vi "GC Vacuum - Step 8.vi"(7 "Step":i32, 8 "error in":errorcluster, 9 "Test Results In":T8, 10 "Gas":T1, 11 "GC Configuration":T2) -> (0 "error out":errorcluster, 1 "Test Results Out":T8, 2 "Gas Out":T1 caption="Gas", 3 "GC Configuration Out":T2)   [LabVIEW 2015]
uses:
  Controls/Test Information.ctl
  Controls/Vacuum Test.ctl
  Controls/Test Timing.ctl
  Controls/Vaccum Thresholds.ctl
  Controls/Helium Test.ctl
  Controls/Helium Thresholds.ctl
  CAN Communication/Gas/Typedefs/Session Handle.ctl
  CAN Communication/Gas/Gas.lvclass
  Controls/Test Results.ctl
  Controls/Step Result.ctl
  CAN Communication/Gas/Typedefs/Valves.ctl
  SubVIs/Timing/Timing.lvlib
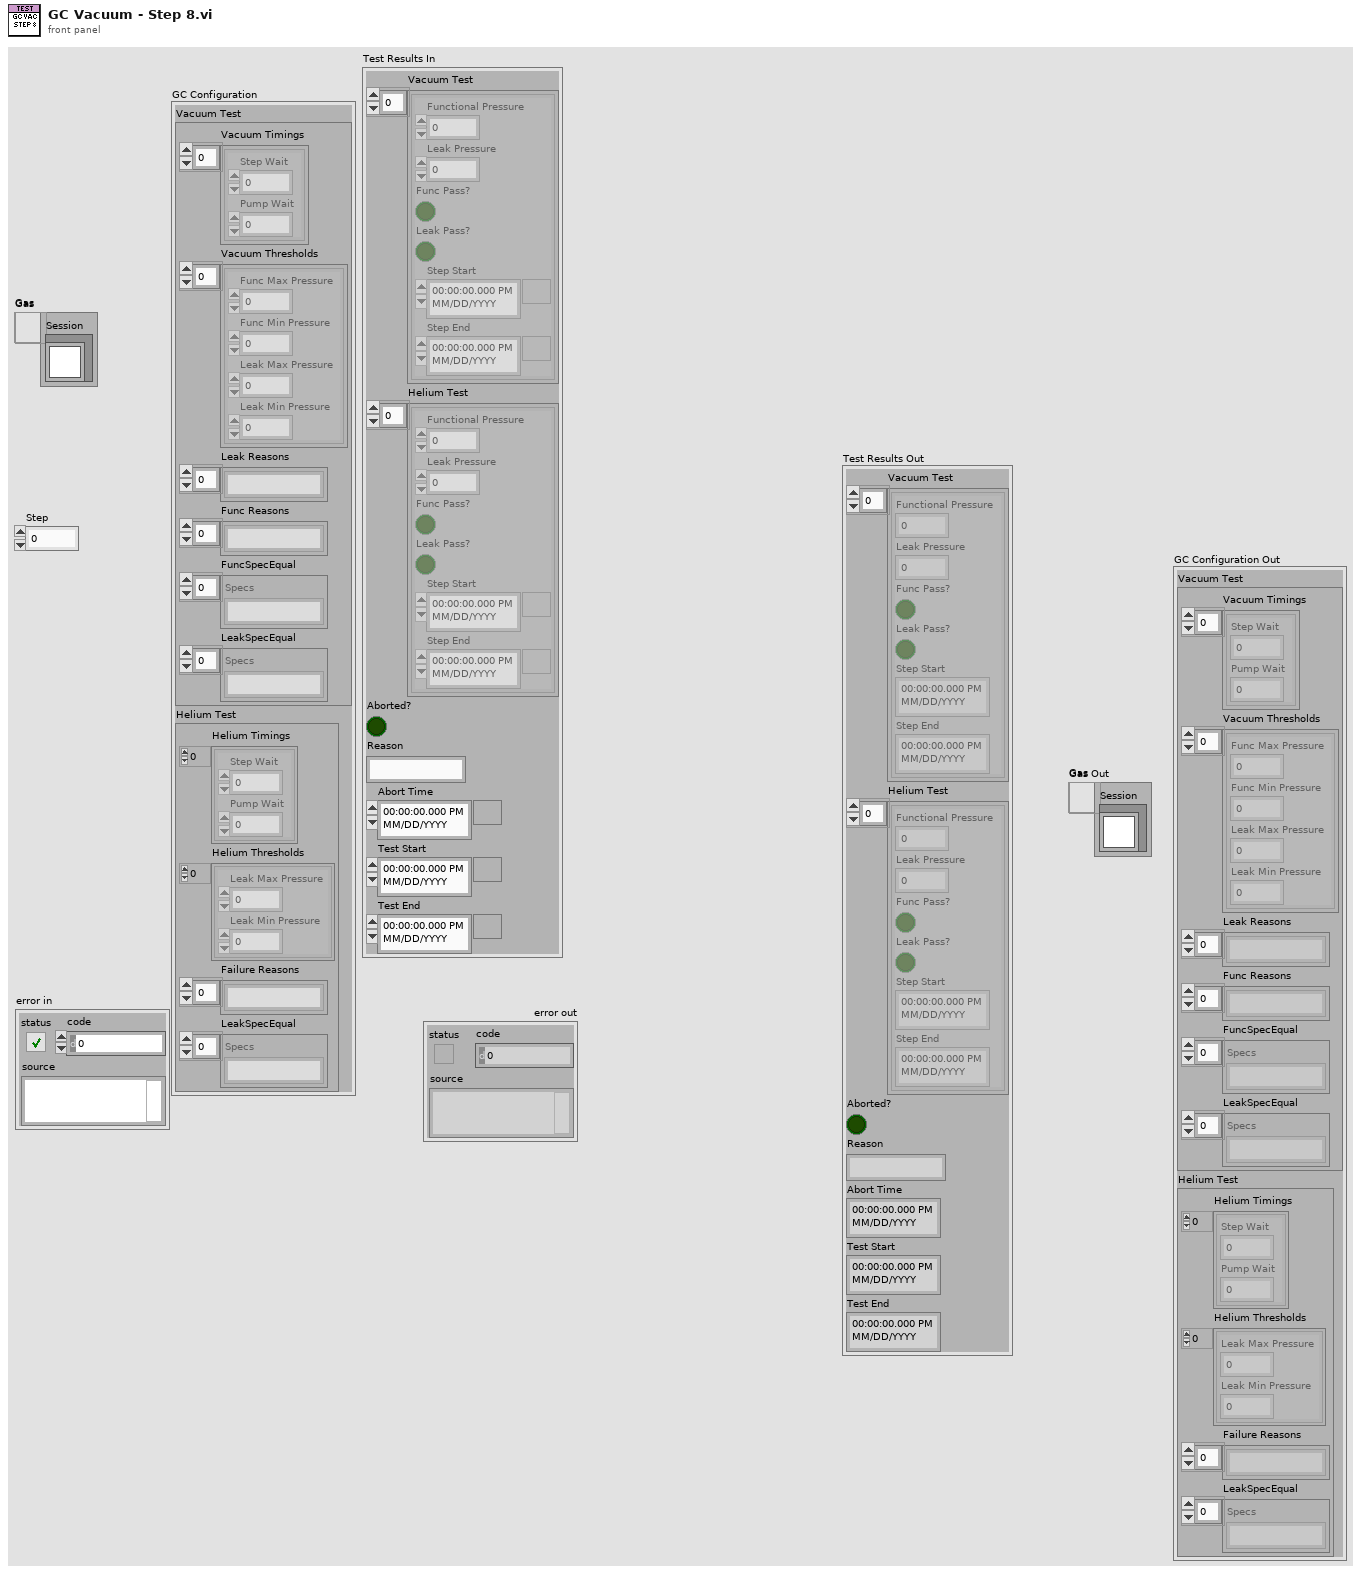
[diagram p1: front panel]
types:
  T1 = typedef "Gas.lvclass/Session Handle.ctl" = refnum<data-value>
  T2 = typedef "Test Information.ctl" = cluster{"Vacuum Test":T3, "Helium Test":T6}
  T3 = typedef "Vacuum Test.ctl" = cluster{"Vacuum Timings":T4[], "Vacuum Thresholds":T5[], "Leak Reasons":string[], "Func Reasons":string[], "FuncSpecEqual":string[], "LeakSpecEqual":string[]}
  T4 = typedef "Test Timing.ctl" = cluster{"Step Wait":dbl, "Pump Wait":dbl}
  T5 = typedef "Vaccum Thresholds.ctl" = cluster{"Func Max Pressure":dbl, "Func Min Pressure":dbl, "Leak Max Pressure":dbl, "Leak Min Pressure":dbl}
  T6 = typedef "Helium Test.ctl" = cluster{"Helium Timings":T4[], "Helium Thresholds":T7[], "Failure Reasons":string[], "LeakSpecEqual":string[]}
  T7 = typedef "Helium Thresholds.ctl" = cluster{"Leak Max Pressure":dbl, "Leak Min Pressure":dbl}
  T8 = typedef "Test Results.ctl" = cluster{"Vacuum Test":T9[], "Helium Test":T9[], "Aborted?":bool, "Reason":string, "Abort Time":timestamp, "Test Start":timestamp, "Test End":timestamp}
  T9 = typedef "Step Result.ctl" = cluster{"Functional Pressure":dbl, "Leak Pressure":dbl, "Func Pass?":bool, "Leak Pass?":bool, "Step Start":timestamp, "Step End":timestamp}
  T10 = typedef "Gas.lvclass/Valves.ctl" = u16
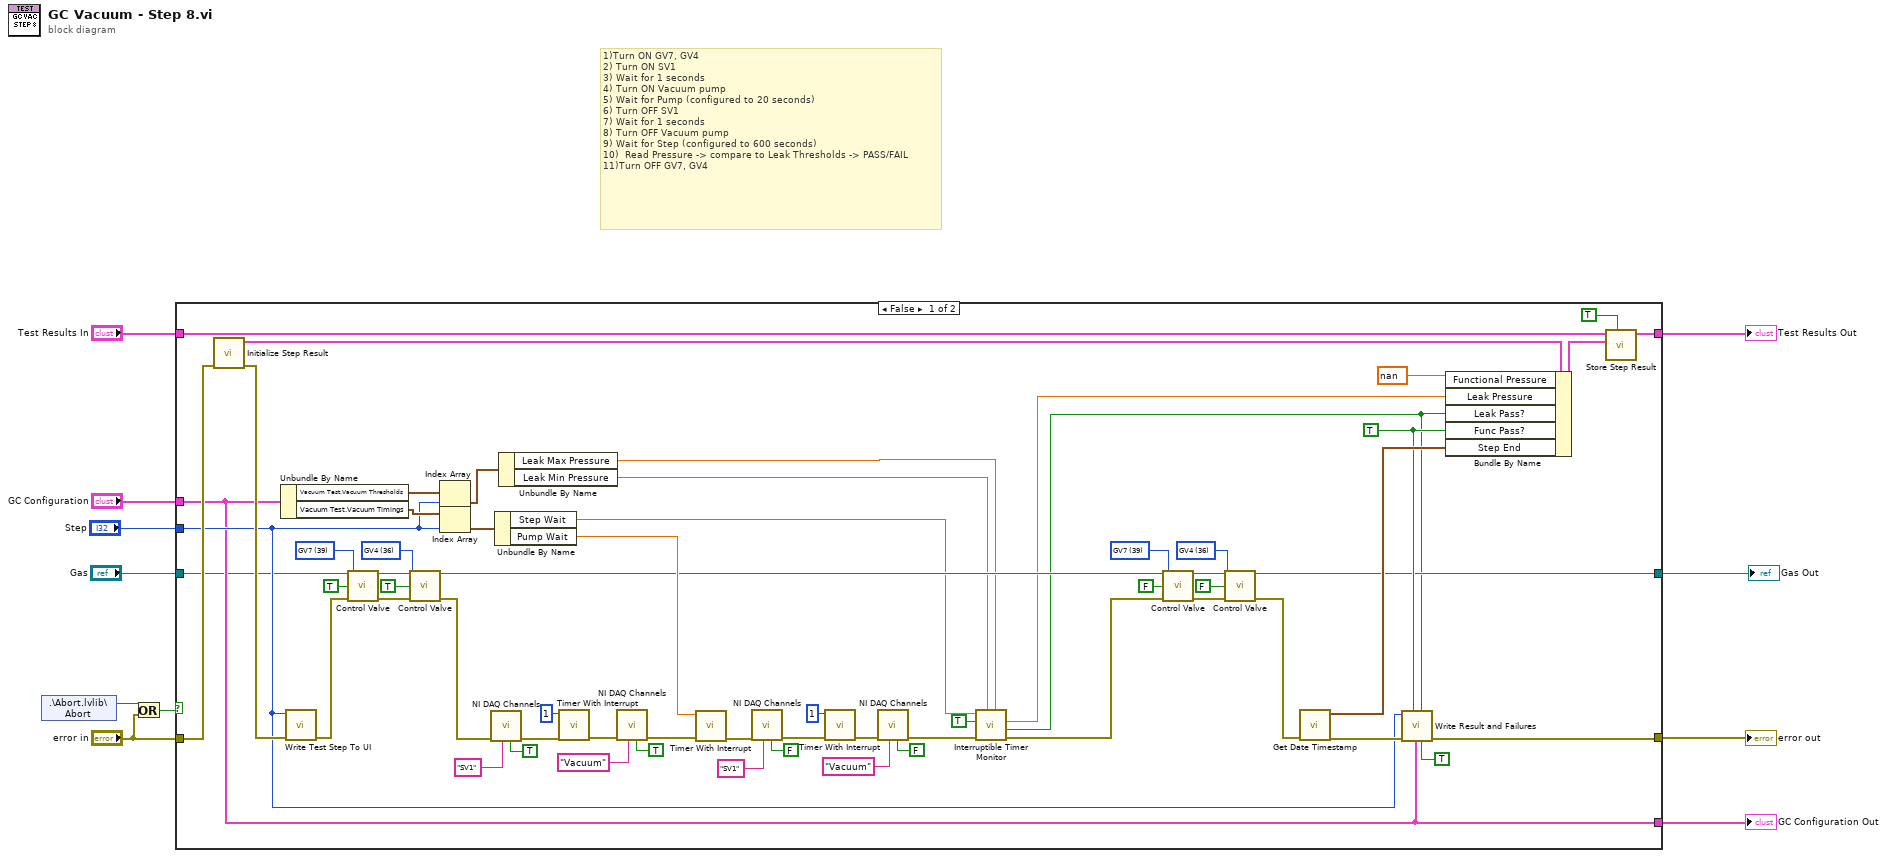
[diagram p0: block diagram]
diagram:
  # "1)Turn ON GV7, GV4\n2) Turn ON SV1\n3) Wait for 1 seconds\n4) Turn ON Vacuum pump\n5) Wait for Pump (configured to 20 seconds)\n6) Turn OFF SV1\n7) Wait for 1 seconds\n8) Turn OFF Vacuum pump\n9) Wait for Step (configured to 600 seconds)\n10)  Read Pressure -> compare to Leak Thresholds -> PASS/FAIL\n11)Turn OFF GV7, GV4"
  n1 = shared-variable ".\\Abort.lvlib\\Abort"() -> (w10:bool)  [unwired: 1 in, 1 out]
  n2 = Or(x=w10, y="error in") -> (x .or. y?=w9:bool)
  n3 = case shown="False" w9 {
    tunnel: "error in" -> [w73 w76]
    tunnel: "Test Results In" -> [w70 w77]
    tunnel: [w71 w77] -> w7
    tunnel: [w61 w76] -> w6
    tunnel: "GC Configuration" -> [w59 w75]
    tunnel: "Step" -> [w60 _]
    tunnel: [w59 w75] -> w3
    tunnel: [w38 w74] -> w1
    tunnel: "Gas" -> [w55 w74]
    frame False {
      w39 = TRUE
      w48 = T10 36 items=["GV1"=33, "GV2"=34, "GV3"=35, "GV4"=36, "GV5"=37, "GV6"=38, "GV7"=39, "GV8"=40, "GV9"=41, "GV10"=42, "GV11"=43, "LV3"=51, "LV4"=52] ("Valves")
      w43 = T10 39 items=["GV1"=33, "GV2"=34, "GV3"=35, "GV4"=36, "GV5"=37, "GV6"=38, "GV7"=39, "GV8"=40, "GV9"=41, "GV10"=42, "GV11"=43, "LV3"=51, "LV4"=52] ("Valves")
      w49 = T10 36 items=["GV1"=33, "GV2"=34, "GV3"=35, "GV4"=36, "GV5"=37, "GV6"=38, "GV7"=39, "GV8"=40, "GV9"=41, "GV10"=42, "GV11"=43, "LV3"=51, "LV4"=52] ("Valves")
      w54 = T10 39 items=["GV1"=33, "GV2"=34, "GV3"=35, "GV4"=36, "GV5"=37, "GV6"=38, "GV7"=39, "GV8"=40, "GV9"=41, "GV10"=42, "GV11"=43, "LV3"=51, "LV4"=52] ("Valves")
      n4 = call "Initialize Step Result.vi"("error in (no error)"=w73) -> ("error out"=w72:errorcluster, "New Step Result"=w69:T9)  [unwired: 8 in, 1 out]
      n5 = Unbundle By Name(w59) -> ("Vacuum Test.Vacuum Thresholds"=w66:T5[], "Vacuum Test.Vacuum Timings"=w65:T4[])
      n6 = call "Write Test Step To UI.vi"("error in (no error)"=w72, "Step"=w60) -> ("error out"=w42:errorcluster)  [unwired: 9 in]
      n7 = call "Control Valve.vi"("Session Handle in"=w55, "Valves"=w54, "Energize?"=TRUE, "error in (no error)"=w42) -> ("Session Handle out"=w50:T1, "error out"=w53:errorcluster)  [unwired: 9 in, 1 out]
      n8 = call "Control Valve.vi"("Session Handle in"=w50, "Valves"=w49, "Energize?"=TRUE, "error in (no error)"=w53) -> ("Session Handle out"=w41:T1, "error out"=w34:errorcluster)  [unwired: 9 in, 1 out]
      n9 = Index Array(array=w66, index=w60) -> (element=w63:T5)
      n10 = Index Array(array=w65, index=w60) -> (element=w64:T4)
      n11 = call "NI DAQ Channels.vi"("Control"=TRUE ("State"), "Channel"="SV1", "error in (no error)"=w34) -> ("error out"=w33:errorcluster)  [unwired: 7 in, 1 out]
      n12 = Unbundle By Name(w64) -> ("Step Wait"=w21:dbl, "Pump Wait"=w57:dbl)
      n13 = Unbundle By Name(w63) -> ("Leak Max Pressure"=w19:dbl, "Leak Min Pressure"=w20:dbl)
      n14 = call "Timer With Interrupt.vi"("error in (no error)"=w33, "Wait (s)"=1) -> ("error out"=w31:errorcluster)  [unwired: 7 in, 2 out]
      n15 = call "NI DAQ Channels.vi"("Control"=TRUE ("State"), "Channel"="Vacuum", "error in (no error)"=w31) -> ("error out"=w30:errorcluster)  [unwired: 7 in, 1 out]
      n16 = call "Timer With Interrupt.vi"("error in (no error)"=w30, "Wait (s)"=w57) -> ("error out"=w28:errorcluster)  [unwired: 7 in, 2 out]
      n17 = call "NI DAQ Channels.vi"("Control"=FALSE ("State"), "Channel"="SV1", "error in (no error)"=w28) -> ("error out"=w27:errorcluster)  [unwired: 7 in, 1 out]
      n18 = call "Timer With Interrupt.vi"("error in (no error)"=w27, "Wait (s)"=1) -> ("error out"=w25:errorcluster)  [unwired: 7 in, 2 out]
      n19 = call "NI DAQ Channels.vi"("Control"=FALSE ("State"), "Channel"="Vacuum", "error in (no error)"=w25) -> ("error out"=w23:errorcluster)  [unwired: 7 in, 1 out]
      n20 = call "Interruptible Timer Monitor.vi"("Max"=w19, "Min"=w20, "error in (no error)"=w23, "Update UI?"=TRUE, "Wait (s)"=w21) -> ("error out"=w22:errorcluster, "In Range?"=w17:bool, "Leak Rate"=w18:dbl)  [unwired: 2 in, 2 out]
      n21 = call "Control Valve.vi"("Session Handle in"=w41, "Valves"=w43, "Energize?"=FALSE, "error in (no error)"=w22) -> ("Session Handle out"=w47:T1, "error out"=w44:errorcluster)  [unwired: 9 in, 1 out]
      n22 = call "Control Valve.vi"("Session Handle in"=w47, "Valves"=w48, "Energize?"=FALSE, "error in (no error)"=w44) -> ("Session Handle out"=w38:T1, "error out"=w37:errorcluster)  [unwired: 9 in, 1 out]
      n23 = call "Get Date Timestamp.vi"("error in (no error)"=w37) -> ("error out"=w62:errorcluster, "current time"=w67:timestamp)  [unwired: 9 in]
      n24 = call "Write Result and Failures.vi"("Vacuum?"=TRUE, "Leak"=w17, "GC Configuration"=w59, "Func"=w39, "error in (no error)"=w62, "Step"=w60) -> ("error out"=w61:errorcluster)  [unwired: 5 in]
      n25 = Bundle By Name(cluster=w69, "Functional Pressure"=nan ("Step Pressure"), "Leak Pressure"=w18, "Leak Pass?"=w17, "Func Pass?"=w39, "Step End"=w67) -> (w68:T9)
      n26 = call "Store Step Result.vi"("Vacuum?"=TRUE, "Step Result"=w68, "Test Results In"=w70) -> ("Test Results Out"=w71:T8)  [unwired: 8 in]
    }
    frame True {
    }
  }
  "error out" <- w6
  "Test Results Out" <- w7
  "GC Configuration Out" <- w3
  "Gas Out" <- w1
